vi "Run Javascript.vi"(5 "Decode Result (T)":bool=TRUE, 7 "Fetch Result (T)":bool=TRUE, 8 "error in (no error)":errorcluster, 10 "javaScript":string, 11 "WebView2 Control in":refnum<class "WebView2 Control.lvclass">) -> (0 "error out":errorcluster, 2 "Result":string, 3 "WebView2 Control out":refnum<class "WebView2 Control.lvclass">)   [LabVIEW 2020, in "WebView2.lvlib" / "WebView2 Control.lvclass"]
uses:
  WebView2 Control.lvclass
  WebView2 Control.lvclass/WebView2 Control.ctl
  C:/Users/Simon/Documents/GitHub/LV-WebView2/Source/Libs/Microsoft.Web.WebView2.Core.dll
  Libs/Microsoft.Web.WebView2.Core.dll
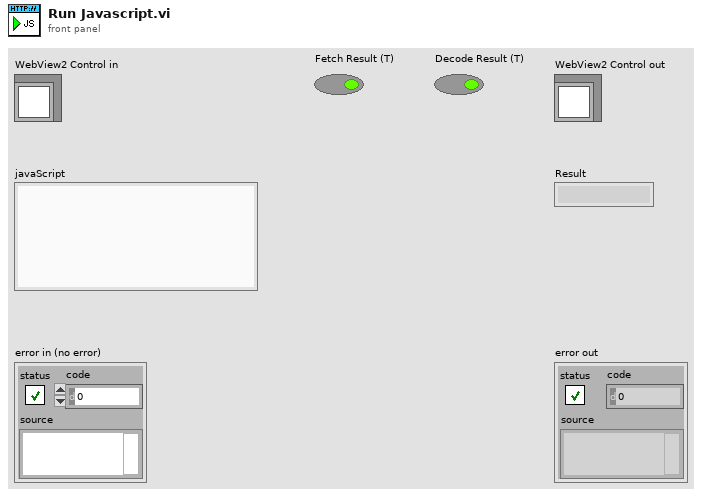
[diagram p1: front panel]
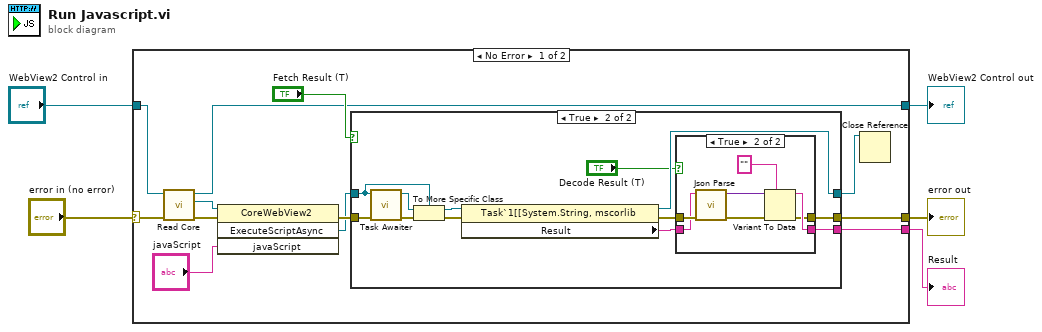
[diagram p0: block diagram]
diagram:
  n1 = case shown="No Error" "error in (no error)" {
    selector: "error in (no error)" -> [w10 w42]
    tunnel: [w11 w42] -> w2
    tunnel: "WebView2 Control in" -> [w8 w41]
    tunnel: [w12 _] -> w1
    tunnel: [w6 w41] -> w3
    frame No Error {
      n2 = call "Read Core.vi"("error in (no error)"=w10, "WebView2.lvlib:WebView2 Control.lvclass"=w8) -> ("error out"=w9:errorcluster, "Webview2 Core"=w7:refnum<k24>, "WebView2.lvlib:WebView2 Control.lvclass"=w6:refnum<class "WebView2 Control.lvclass">)  [unwired: 7 in]
      n3 = invoke class="CoreWebView2" method="ExecuteScriptAsync"(reference=w7, error in=w9, "javaScript"="javaScript") -> (error out=w14:errorcluster, "ExecuteScriptAsync"=w13:refnum<k24>)  [unwired: 1 in, 2 out]
      n4 = case shown="True" "Fetch Result (T)" {
        tunnel: w13 -> [w18 w22]
        tunnel: w14 -> [w19 w20]
        tunnel: [w18 w31] -> w15
        tunnel: [_ w30] -> w12
        tunnel: [w19 w29] -> w11
        frame False {
        }
        frame True {
          n5 = call "Task Awaiter.vi"("error in (no error)"=w20, "Task"=w22) -> ("error out"=w25:errorcluster, "Task"=w23:refnum<k24>)  [unwired: 7 in, 1 out]
          n6 = To More Specific Class(target class=w22, reference=w23, error in=w25) -> (specific class reference=w21:refnum<k24>, error out=w24:errorcluster)
          n7 = property class="Task`1[[System.String, mscorlib"(reference=w21, error in=w24) -> (reference out=w31:refnum<k24>, error out=w28:errorcluster, "Result"=w27:string)
          n8 = case shown="True" "Decode Result (T)" {
            tunnel: [w33 w39] -> w30
            tunnel: [w32 w38] -> w29
            tunnel: w28 -> [w32 w37]
            tunnel: w27 -> [w33 w36]
            frame False {
            }
            frame True {
              n9 = call "Json Parse.vi"("error in (no error)"=w37, "JSON"=w36) -> ("error out"=w35:errorcluster, "variant"=w34:variant)  [unwired: 8 in]
              n10 = Variant To Data(error in=w35, type="", Variant=w34) -> (data=w39:string, error out=w38:errorcluster)
            }
          }
        }
      }
      n11 = Close Reference(reference=w15) -> ()  [unwired: 1 in, 1 out]
    }
    frame Error {
    }
  }
  "error out" <- w2
  "WebView2 Control out" <- w3
  "Result" <- w1
